vi "Connection Mode Generation Search for Connection (Local Message).vi"(0 "Connections":T2[](array[typedef]) {"Packets"."Identifier" format="%08x"}, 5 "Data to Send":T1 {"Identifier" format="%08x"}, 11 "error in (no error)":errorcluster) -> (4 "Connection Cluster":T2 {"Packets"."Identifier" format="%08x"}, 6 "CAN Frame Out":T1 {"Identifier" format="%08x"}, 8 "Found?":bool, 10 "Index":i32, 15 "error out":errorcluster)   [LabVIEW 2013, in "J1939 Addon Engine.lvlib"]
uses:
  Engine/J1939 Addon Engine.lvlib
  Types/Connection Mode Generation Connection Cluster.ctl
  J1939 Utilities/Types/CAN Outgoing Message Cluster.ctl
  J1939 Utilities/SubVIs/Convert CAN Arb ID to J1939 ID.vi
  J1939 Utilities/J1939 Utilities.lvlib
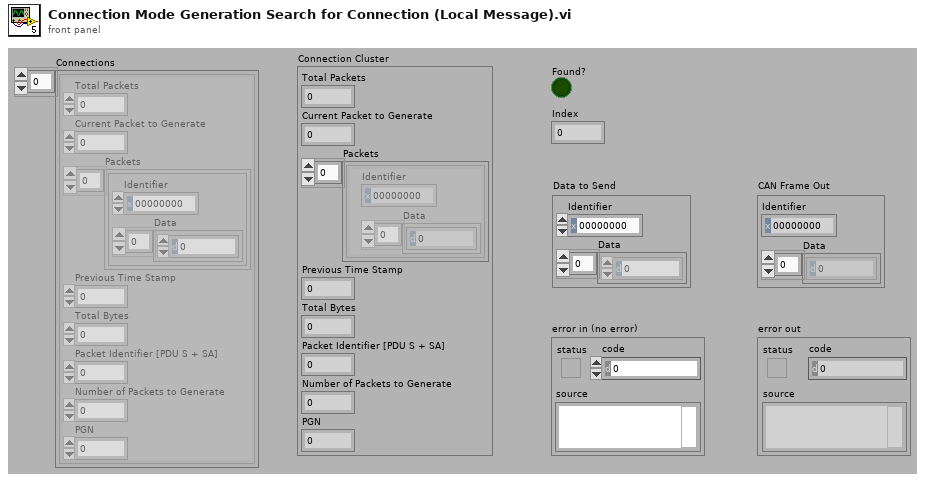
[diagram p1: front panel]
types:
  T1 = typedef "J1939 Utilities.lvlib/CAN Outgoing Message Cluster.ctl" = cluster{"Identifier":u32, "Data":u8[]}
  T2 = typedef "J1939 Addon Engine.lvlib/Connection Mode Generation Connection Cluster.ctl" = cluster{"Total Packets":u8, "Current Packet to Generate":u8, "Packets":T1[], "Previous Time Stamp":u32, "Total Bytes":u16, "Packet Identifier [PDU S + SA]":u16, "Number of Packets to Generate":u8, "PGN":u32}
  T3 = typedef "J1939 Utilities.lvlib/PGN Fields Cluster.ctl" = cluster{"Reserved Bit":u8, "Data page":u8, "PDU Format":u8, "PDU Specific":u8}
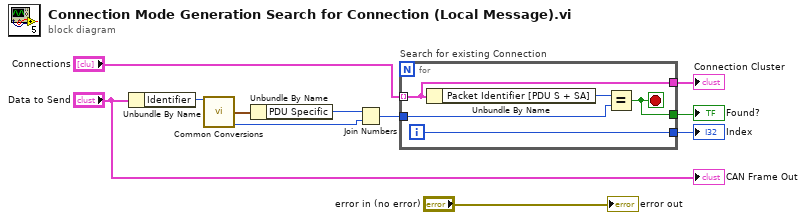
[diagram p0: block diagram]
diagram:
  n1 = Unbundle By Name("Data to Send") -> ("Identifier"=w1:u32)
  n2 = call-poly "Common Conversions.vi"("Arb ID"=w1) -> ("PGN Fields"=w11:T3, "Source Address"=w8:u8)  [unwired: 13 out]
  n3 = Unbundle By Name(w11) -> ("PDU Specific"=w9:u8)
  n4 = Join Numbers(hi=w9, lo=w8) -> ((hi.lo)=w10:u16)
  n5 = for "Search for existing Connection" {
    tunnel: "Connections" -> [w12] mode=indexing
    tunnel: [w15] -> w5
    tunnel: w10 -> [w14]
    tunnel: [w13] -> w4
    tunnel: [w12] -> w6
    i -> [w13]
    stop <- w15 stop-if-true
    n6 = Unbundle By Name(w12) -> ("Packet Identifier [PDU S + SA]"=w16:u16)
    n7 = Equal?(x=w16, y=w14) -> (x = y?=w15:bool)
  }
  "Connection Cluster" <- w6
  "Found?" <- w5
  "Index" <- w4
  "error out" <- "error in (no error)"
  "CAN Frame Out" <- "Data to Send"
